vi "Poly_fit_Special.vi"(4 "polynomial order":i32=2, 5 "Input X^3":dbl[](array[numeric]) format="%.3f", 6 "Point selector":cluster{"Y":dbl, "X":dbl, "switch":bool}[](array[cluster]) {"X" format="%.2f"; "Y" format="%.2f"}, 7 "Input X^2":dbl[](array[numeric]) format="%.3f", 8 "Input X array":dbl[](array[numeric]) format="%.3f", 9 "Input Y array":dbl[](array[numeric]) format="%.4f") -> (0 "Point selector":cluster{"Y":dbl, "X":dbl, "switch":bool}[](array[cluster]) {"X" format="%.2f"; "Y" format="%.2f"}, 1 "Calibration plot":cluster{cluster{dbl, dbl}[]}[](graph), 2 "Coefficients":dbl[](array[numeric]) format="%.2f", 3 "Calib const":string[][](array[string]))   [LabVIEW 2010]
uses:
  <vilib>/Analysis/NI_AALBase.lvlib
  <vilib>/Analysis/NI_AALPro.lvlib
panel:
  out "Array":dbl[][](array[numeric])
  in  "Type":cluster{"Y":dbl, "X":dbl, "switch":bool}={"Y"=10.144154930121, "X"=9.20412, "switch"=FALSE} {"X" format="%.2f"; "Y" format="%.2f"}
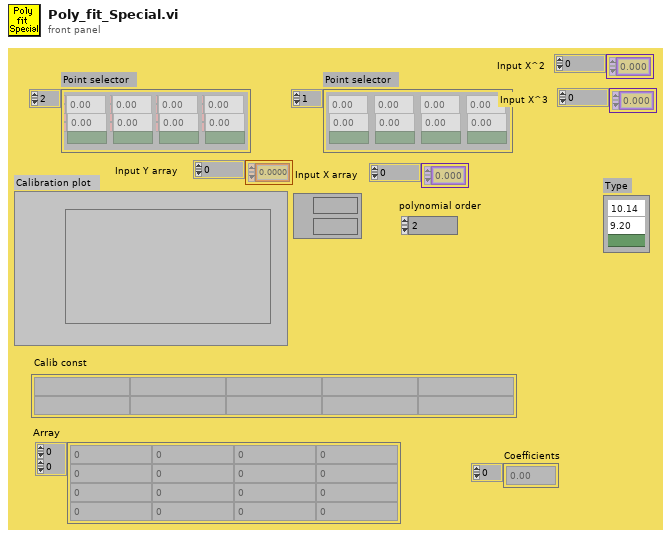
[diagram p1: front panel]
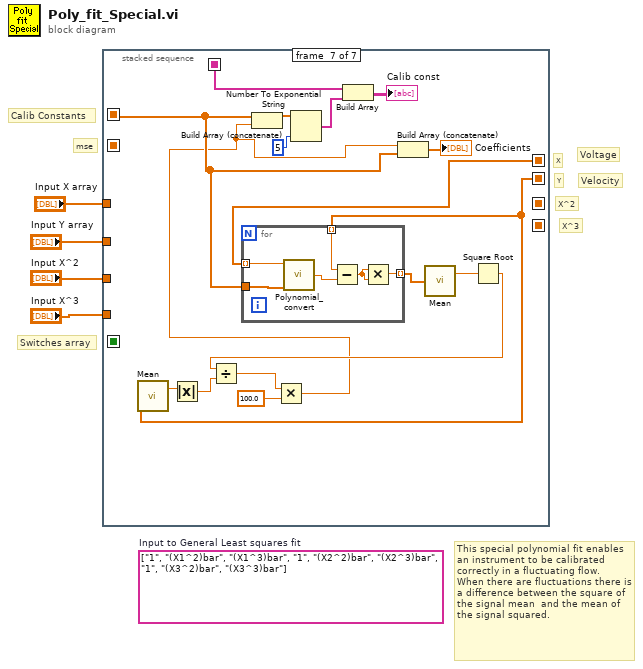
[diagram p0: block diagram]
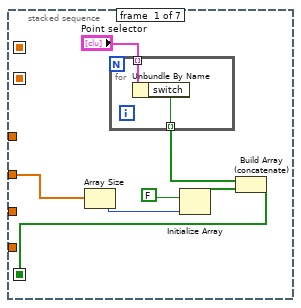
[diagram p2: hidden frame]
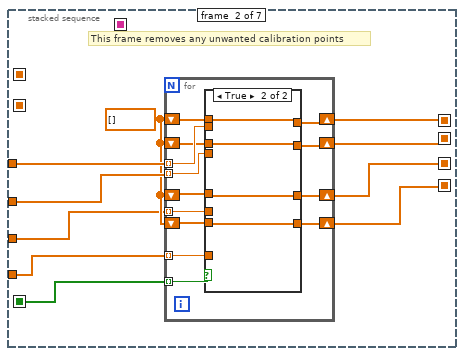
[diagram p3: hidden frame]
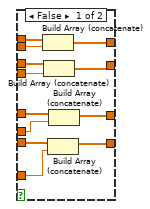
[diagram p4: hidden frame]
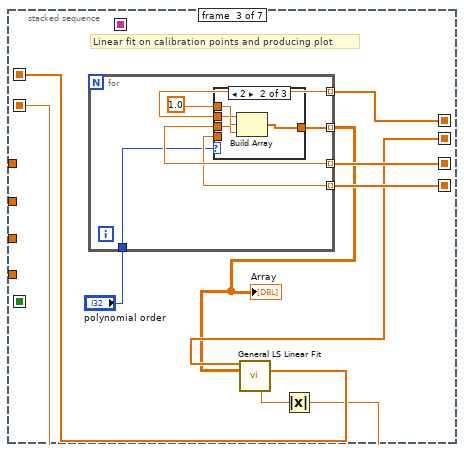
[diagram p5: hidden frame]
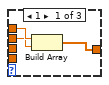
[diagram p6: hidden frame]
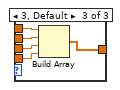
[diagram p7: hidden frame]
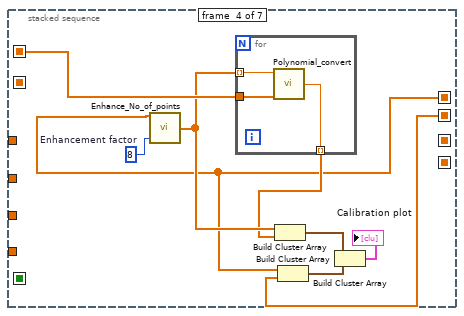
[diagram p8: hidden frame]
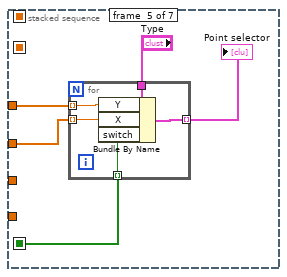
[diagram p9: hidden frame]
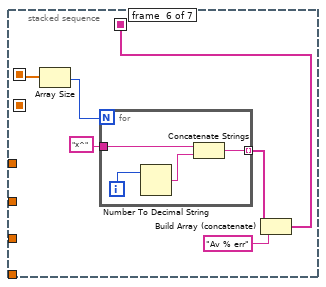
[diagram p10: hidden frame]
diagram:
  (unwired) string[][] [["1", "(X1^2)bar", "(X1^3)bar"], ["1", "(X2^2)bar", "(X2^3)bar"], ["1", "(X3^2)bar", "(X3^3)bar"]]  # Input to General Least squares fit
  # "This special polynomial fit enables an instrument to be calibrated correctly in a fluctuating flow.  When there are fluctuations there is a difference between the square of the signal mean  and the mean of the signal squared."
  # "X^3"
  # "X^2"
  # "mse"
  # "Calib Constants"
  # "Voltage"
  # "Velocity"
  # "Switches array"
  # "X"
  # "Y"
  n1 = stacked-sequence {
    seq-local: [_ w23 _ _ _ _ _] -> [_ _ w61 w81 _ _ w120]
    seq-local: [_ w22 _ _ _ _ _] -> [_ _ w57 w80 _ _ w119]
    seq-local: [w9 _ _ _ _ _ _] -> [_ w19 _ _ w93 _ _]
    seq-local: [_ _ w55 _ _ _ _] -> [_ _ _ w84 _ w105 w121]
    seq-local: [_ _ w53 _ _ _ _] -> [_ _ _ _ _ _ _]
    seq-local: [_ _ _ _ _ w102 _] -> [_ _ _ _ _ _ w125]
    seq-local: [_ w15 _ _ _ _ _] -> [_ _ w60 _ _ _ _]
    seq-local: [_ w14 _ _ _ _ _] -> [_ _ w59 _ _ _ _]
    tunnel: "Input Y array" -> [w5 w20 _ _ w94 _ _]
    tunnel: "Input X array" -> [_ w21 _ _ w95 _ _]
    tunnel: "Input X^2" -> [_ w17 _ _ _ _ _]
    tunnel: "Input X^3" -> [_ w16 _ _ _ _ _]
    frame #0 {
      n2 = Array Size(array=w5) -> (size(s)=w7:i32)
      n3 = for {
        tunnel: "Point selector" -> [w13] mode=indexing
        tunnel: [w12] -> w10 mode=indexing
        n4 = Unbundle By Name(w13) -> ("switch"=w12:bool)
      }
      n5 = Initialize Array(FALSE, w7) -> (w6:bool[])
      n6 = Build Array (concatenate)(w10, w6) -> (w9:bool[])
    }
    frame #1 {
      w18 = dbl[] []
      # "This frame removes any unwanted calibration points"
      n7 = for {
        shift-right: [w30] -> w22
        shift-left: w18 -> [w32]
        shift-right: [w31] -> w23
        shift-left: w18 -> [w33]
        tunnel: w19 -> [w34] mode=indexing
        tunnel: w20 -> [w35] mode=indexing
        tunnel: w21 -> [w36] mode=indexing
        shift-right: [w24] -> w15
        shift-left: w18 -> [w29]
        shift-right: [w25] -> w14
        shift-left: w18 -> [w28]
        tunnel: w17 -> [w27] mode=indexing
        tunnel: w16 -> [w26] mode=indexing
        n8 = case shown="True" w34 {
          tunnel: [w43 w51] -> w30
          tunnel: [w44 w52] -> w31
          tunnel: w32 -> [w45 w51]
          tunnel: w33 -> [w46 w52]
          tunnel: w35 -> [w47 _]
          tunnel: w36 -> [w48 _]
          tunnel: w29 -> [w42 w50]
          tunnel: w28 -> [w41 w49]
          tunnel: w27 -> [w40 _]
          tunnel: w26 -> [w39 _]
          tunnel: [w38 w49] -> w25
          tunnel: [w37 w50] -> w24
          frame False {
            n9 = Build Array (concatenate)(w46, w48) -> (w44:dbl[])
            n10 = Build Array (concatenate)(w45, w47) -> (w43:dbl[])
            n11 = Build Array (concatenate)(w41, w39) -> (w38:dbl[])
            n12 = Build Array (concatenate)(w42, w40) -> (w37:dbl[])
          }
          frame True {
          }
        }
      }
    }
    frame #2 {
      # "Linear fit on calibration points and producing plot"
      n13 = for {
        tunnel: w61 -> [w66] mode=indexing
        tunnel: w60 -> [w65] mode=indexing
        tunnel: w59 -> [w64] mode=indexing
        tunnel: "polynomial order" -> [w63]
        tunnel: [w62] -> w54 mode=indexing
        n14 = case shown="2" w63 {
          tunnel: 1.0 -> [w70 w74 w79]
          tunnel: w66 -> [w69 w73 w78]
          tunnel: w65 -> [_ w72 w77]
          tunnel: w64 -> [_ _ w76]
          tunnel: [w68 w71 w75] -> w62
          frame 1 {
            n15 = Build Array(w70, w69) -> (w68:dbl[])
          }
          frame 2 {
            n16 = Build Array(w74, w73, w72) -> (w71:dbl[])
          }
          frame 3, Default {
            n17 = Build Array(w79, w78, w77, w76) -> (w75:dbl[])
          }
        }
      }
      "Array" <- w54
      n18 = call <vilib>:"General LS Linear Fit.vi"("Y"=w57, "H"=w54) -> ("Coefficients"=w55:dbl[], "mse"=w56:dbl)  [unwired: 3 in, 9 out]
      n19 = Absolute Value(x=w56) -> (abs(x)=w53:dbl)
    }
    frame #3 {
      w85 = 8  # Enhancement factor
      n20 = call "Enhance_No_of_points.vi"("Enhancement factor"=w85, "Input"=w81) -> ("Output"=w83:dbl[])  [unwired: 3 out]
      n21 = for {
        tunnel: w84 -> [w91]
        tunnel: w83 -> [w90] mode=indexing
        tunnel: [w89] -> w82 mode=indexing
        n22 = call "Polynomial_convert.vi"("Calib constants"=w91, "Voltage"=w90) -> ("Eng Values"=w89:dbl)  [unwired: 4 out]
      }
      n23 = Build Cluster Array(w83, w82) -> (w88:cluster{dbl, "Eng Values":dbl}[])
      n24 = Build Cluster Array(w81, w80) -> (w87:cluster{dbl, dbl}[])
      n25 = Build Cluster Array(w88, w87) -> (→"Calibration plot":cluster{cluster{dbl, "Eng Values":dbl}[]}[])
    }
    frame #4 {
      n26 = for {
        tunnel: "Type" -> [w101]
        tunnel: w95 -> [w100] mode=indexing
        tunnel: w94 -> [w99] mode=indexing
        tunnel: w93 -> [w98] mode=indexing
        tunnel: [w97] -> w92 mode=indexing
        n27 = Bundle By Name(cluster=w101, "Y"=w100, "X"=w99, "switch"=w98) -> (w97:cluster{"Y":dbl, "X":dbl, "switch":bool})
      }
      "Point selector" <- w92
    }
    frame #5 {
      n28 = Array Size(array=w105) -> (size(s)=w104:i32)
      n29 = for {
        N: w104 -> [_]
        tunnel: "x^" -> [w109]
        tunnel: [w108] -> w103 mode=indexing
        i -> [w111]
        n30 = Number To Decimal String(number=w111) -> (decimal integer string=w110:string)  [unwired: 1 out]
        n31 = Concatenate Strings(w109, w110) -> (w108:string)
      }
      n32 = Build Array (concatenate)(w103, "Av % err") -> (w102:string[])
    }
    frame #6 {
      n33 = call <vilib>:"Mean.vi"("X"=w119) -> ("mean"=w122:dbl)  [unwired: 1 out]
      n34 = Absolute Value(x=w122) -> (abs(x)=w116:dbl)
      n35 = for {
        tunnel: w121 -> [w134]
        tunnel: w120 -> [w133] mode=indexing
        tunnel: w119 -> [w131] mode=indexing
        tunnel: [w129] -> w113 mode=indexing
        n36 = call "Polynomial_convert.vi"("Calib constants"=w134, "Voltage"=w133) -> ("Eng Values"=w132:dbl)  [unwired: 4 out]
        n37 = Subtract(x=w131, y=w132) -> (x-y=w130:dbl)
        n38 = Multiply(x=w130, y=w130) -> (x*y=w129:dbl)
      }
      n39 = call <vilib>:"Mean.vi"("X"=w113) -> ("mean"=w112:dbl)  [unwired: 1 out]
      n40 = Square Root(x=w112) -> (sqrt(x)=w117:dbl)
      n41 = Divide(x=w117, y=w116) -> (x/y=w115:dbl)
      n42 = Multiply(x=w115, y=100.0) -> (x*y=w114:dbl)
      n43 = Build Array (concatenate)(w121, w114) -> (w128:dbl[])
      n44 = Number To Exponential String(number=w128, precision (6)=i16 5) -> (E-format string=w127:string[])  [unwired: 2 out]
      n45 = Build Array(w125, w127) -> (→"Calib const":string[][])
      n46 = Build Array (concatenate)(w114, w121) -> (→"Coefficients":dbl[])
    }
  }
